vi "UpdateDB_PV.vi"(5 "Trace name":string, 7 "Process name":string, 8 "error in (no error)":errorcluster, 9 "Time Stamp":timestamp, 10 "Double":dbl, 11 "database URL":path) -> (0 "error out":errorcluster)   [LabVIEW 2013]
uses:
  <vilib>/lvdsc/historical/Open Trace (Numeric).vi
  <vilib>/lvdsc/historical/Write Trace (Numeric).vi
  <vilib>/lvdsc/NI_DSC.lvlib
panel:
  out "x < y?":bool
  out "x-y":dbl
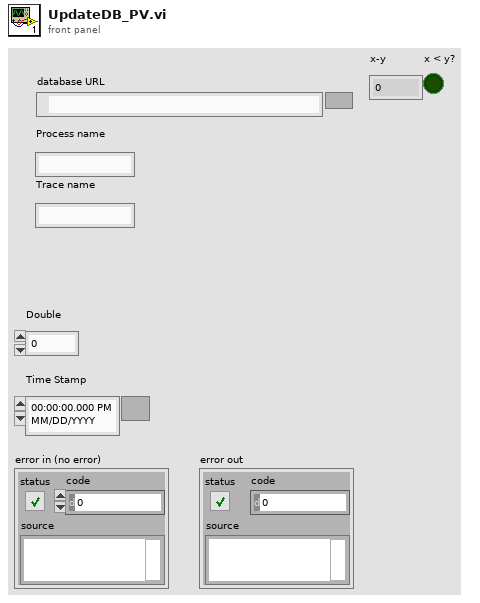
[diagram p1: front panel]
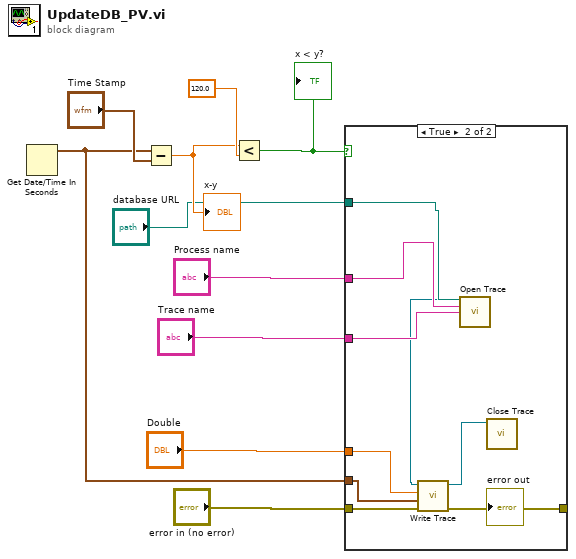
[diagram p0: block diagram]
diagram:
  n1 = Get Date/Time In Seconds() -> (seconds since 1Jan1904=w1:timestamp)
  n2 = Subtract(x=w1, y="Time Stamp") -> (x-y=w5:dbl)
  "x-y" <- w5
  n3 = Less?(x=w5, y=120.0 ("x")) -> (x < y?=w10:bool)
  "x < y?" <- w10
  n4 = case shown="True" w10 {
    tunnel: "error in (no error)" -> [w11 w20]
    tunnel: [w11 w19] -> _
    tunnel: "Double" -> [_ w18]
    tunnel: "database URL" -> [_ w17]
    tunnel: "Process name" -> [_ w16]
    tunnel: "Trace name" -> [_ w15]
    tunnel: w1 -> [_ w12]
    frame False {
    }
    frame True {
      n5 = call-poly <vilib>:"Open Trace.vi"("database URL"=w17, "process name"=w16, "trace name"=w15) -> ("trace reference"=w13:refnum<k1>)  [unwired: 10 in, 2 out]
      n6 = call-poly <vilib>:"Write Trace.vi"("error in (no error)"=w20, "timestamp (now)"=w12, "value"=w18, "trace ref"=w13) -> ("error out"=w19:errorcluster, "trace ref out"=w14:refnum<k1>)  [unwired: 6 in]
      n7 = call <vilib>:"Close Trace.vi"("trace reference"=w14) -> ()  [unwired: 10 in, 1 out]
    }
  }
